vi "Acquire channel.vi"(8 "error in (no error)":errorcluster, 9 "Channel":i32, 10 "Acquisition cluster":T2, 11 "Instrument cluster":T1) -> (0 "error out":errorcluster, 2 "Image Array":u16[][](array[numeric]))   [LabVIEW 2017]
uses:
  C:/Program Files/National Instruments/LabVIEW 2017/instr.lib/IDS/ueye.NET/uEyeDotNet.dll
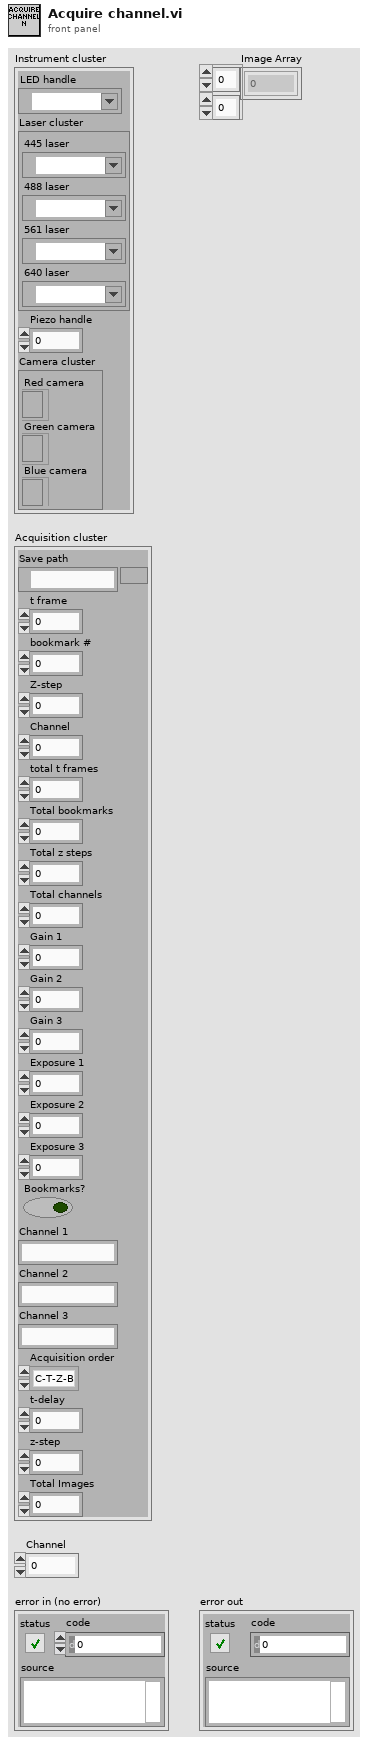
[diagram p1: front panel]
types:
  T1 = cluster{"LED handle":refnum<visa-resource-name>, "Laser cluster":cluster{"445 laser":refnum<visa-resource-name>, "488 laser":refnum<visa-resource-name>, "561 laser":refnum<visa-resource-name>, "640 laser":refnum<visa-resource-name>}, "Piezo handle":i32, "Camera cluster":cluster{"Red camera":refnum<k24>, "Green camera":refnum<k24>, "Blue camera":refnum<k24>}}
  T2 = cluster{"Save path":path, "t frame":i32, "bookmark #":i32, "Z-step":i32, "Channel":i32, "total t frames":i32, "Total bookmarks":i32, "Total z steps":i32, "Total channels":i32, "Gain 1":i32, "Gain 2":i32, "Gain 3":i32, "Exposure 1":dbl, "Exposure 2":dbl, "Exposure 3":dbl, "Bookmarks?":bool, "Channel 1":string, "Channel 2":string, "Channel 3":string, "Acquisition order":enum16{"C-T-Z-B", "C-T-B-Z", "C-Z-T-B", "C-Z-B-T", "C-B-T-Z", "C-B-Z-T", "T-C-Z-B", "T-C-B-Z", "T-Z-C-B", "T-Z-B-C", "T-B-C-Z", "T-B-Z-C", "Z-C-T-B", "Z-C-B-T", "Z-T-C-B", "Z-T-B-C", "Z-B-C-T", "Z-B-T-C", "B-C-T-Z", "B-C-Z-T", "B-Z-C-T", "B-Z-T-C", "B-T-C-Z", "B-T-Z-C"}, "t-delay":dbl, "z-step":dbl, "Total Images":i32}
  T3 = cluster{"445 laser":refnum<visa-resource-name>, "488 laser":refnum<visa-resource-name>, "561 laser":refnum<visa-resource-name>, "640 laser":refnum<visa-resource-name>}
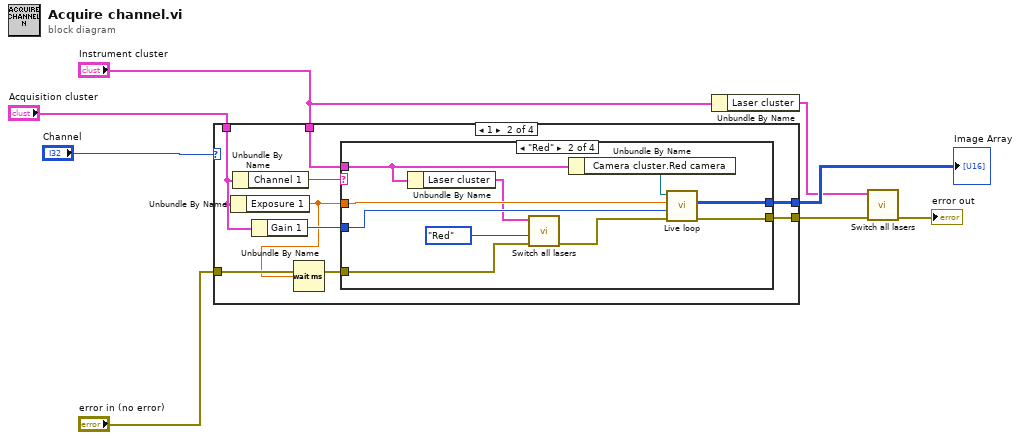
[diagram p0: block diagram]
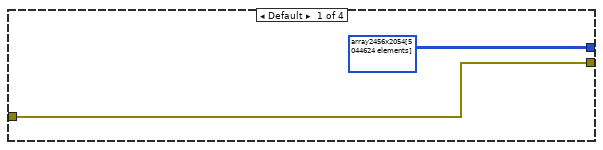
[diagram p2: hidden frame]
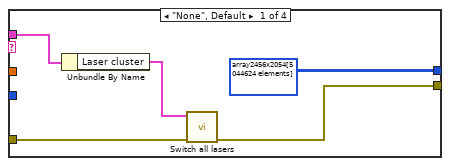
[diagram p3: hidden frame]
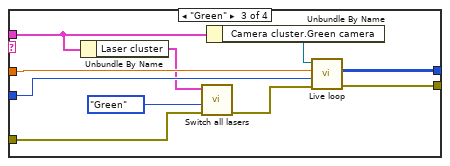
[diagram p4: hidden frame]
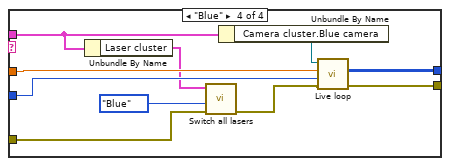
[diagram p5: hidden frame]
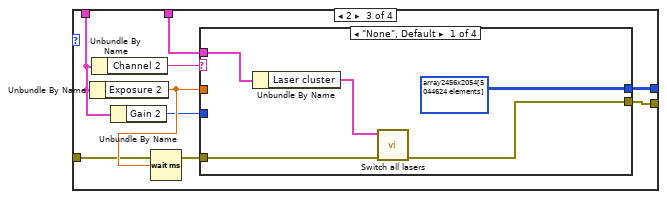
[diagram p6: hidden frame]
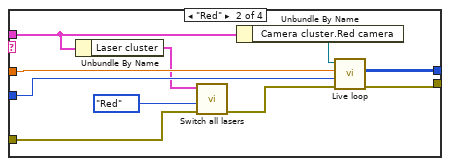
[diagram p7: hidden frame]
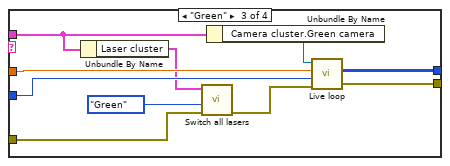
[diagram p8: hidden frame]
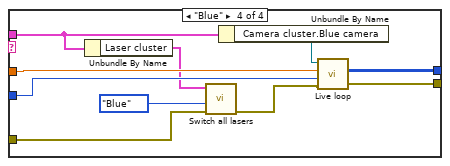
[diagram p9: hidden frame]
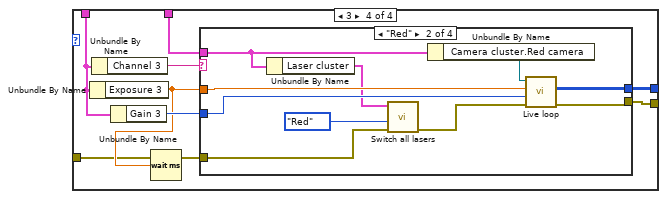
[diagram p10: hidden frame]
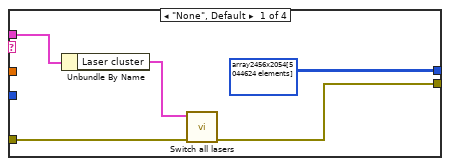
[diagram p11: hidden frame]
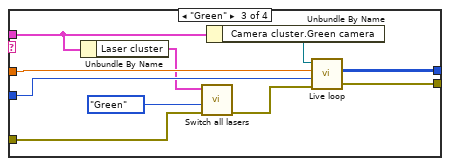
[diagram p12: hidden frame]
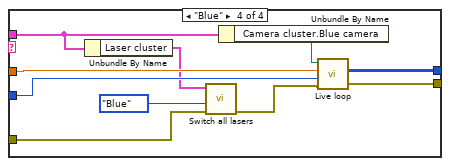
[diagram p13: hidden frame]
diagram:
  n1 = case shown="1" "Channel" {
    tunnel: "Acquisition cluster" -> [_ w17 w61 w104]
    tunnel: "Instrument cluster" -> [_ w16 w59 w101]
    tunnel: "error in (no error)" -> [w10 w14 w55 w97]
    tunnel: [w10 w12 w60 w103] -> w4
    tunnel: [u16[][] array2456x2054[5044624 elements] ("Image Array") w11 w54 w102] -> w6
    frame Default {
    }
    frame 1 {
      n2 = Unbundle By Name(w17) -> ("Exposure 1"=w13:dbl)
      n3 = Unbundle By Name(w17) -> ("Channel 1"=w18:string)
      n4 = Unbundle By Name(w17) -> ("Gain 1"=w15:i32)
      n5 = Wait (ms)(milliseconds to wait=w13) -> ()  [unwired: 1 out]
      n6 = case shown="\"Red\"" w18 {
        tunnel: w16 -> [w19 w25 w36 w45]
        tunnel: w15 -> [_ w33 w43 w53]
        tunnel: w13 -> [_ w32 w42 w52]
        tunnel: w14 -> [w21 w28 w35 w44]
        tunnel: [w20 w29 w39 w49] -> w12
        tunnel: [u16[][] array2456x2054[5044624 elements] ("Image Array") w30 w40 w50] -> w11
        frame "None", Default {
          n7 = Unbundle By Name(w19) -> ("Laser cluster"=w22:T3)
          n8 = call "Switch all lasers.vi"("error in"=w21, "Laser cluster"=w22) -> ("error out"=w20:errorcluster)  [unwired: 9 in]
        }
        frame "Red" {
          n9 = Unbundle By Name(w25) -> ("Laser cluster"=w24:T3)
          n10 = call "Switch all lasers.vi"("error in"=w28, "Live channel"=enum8{"Red", "Green", "Blue", ""}."Red", "Laser cluster"=w24) -> ("error out"=w27:errorcluster)  [unwired: 8 in]
          n11 = Unbundle By Name(w25) -> ("Camera cluster.Red camera"=w31:refnum<k24>)
          n12 = call "Live loop.vi"("Error In"=w27, "Gain"=w33, "Exposure time (ms)"=w32, "Camera reference in"=w31) -> ("Error Out"=w29:errorcluster, "Image Array"=w30:u16[][])  [unwired: 4 in, 1 out]
        }
        frame "Green" {
          n13 = Unbundle By Name(w36) -> ("Laser cluster"=w38:T3)
          n14 = call "Switch all lasers.vi"("error in"=w35, "Live channel"=enum8{"Red", "Green", "Blue", ""}."Green", "Laser cluster"=w38) -> ("error out"=w34:errorcluster)  [unwired: 8 in]
          n15 = Unbundle By Name(w36) -> ("Camera cluster.Green camera"=w41:refnum<k24>)
          n16 = call "Live loop.vi"("Error In"=w34, "Gain"=w43, "Exposure time (ms)"=w42, "Camera reference in"=w41) -> ("Error Out"=w39:errorcluster, "Image Array"=w40:u16[][])  [unwired: 4 in, 1 out]
        }
        frame "Blue" {
          n17 = Unbundle By Name(w45) -> ("Laser cluster"=w48:T3)
          n18 = call "Switch all lasers.vi"("error in"=w44, "Live channel"=enum8{"Red", "Green", "Blue", ""}."Blue", "Laser cluster"=w48) -> ("error out"=w46:errorcluster)  [unwired: 8 in]
          n19 = Unbundle By Name(w45) -> ("Camera cluster.Blue camera"=w51:refnum<k24>)
          n20 = call "Live loop.vi"("Error In"=w46, "Gain"=w53, "Exposure time (ms)"=w52, "Camera reference in"=w51) -> ("Error Out"=w49:errorcluster, "Image Array"=w50:u16[][])  [unwired: 4 in, 1 out]
        }
      }
    }
    frame 2 {
      n21 = Unbundle By Name(w61) -> ("Exposure 2"=w57:dbl)
      n22 = Unbundle By Name(w61) -> ("Channel 2"=w58:string)
      n23 = Unbundle By Name(w61) -> ("Gain 2"=w56:i32)
      n24 = Wait (ms)(milliseconds to wait=w57) -> ()  [unwired: 1 out]
      n25 = case shown="\"None\", Default" w58 {
        tunnel: w59 -> [w62 w68 w79 w88]
        tunnel: w56 -> [_ w76 w86 w96]
        tunnel: w57 -> [_ w75 w85 w95]
        tunnel: w55 -> [w64 w71 w78 w87]
        tunnel: [w63 w72 w82 w92] -> w60
        tunnel: [u16[][] array2456x2054[5044624 elements] ("Image Array") w73 w83 w93] -> w54
        frame "None", Default {
          n26 = Unbundle By Name(w62) -> ("Laser cluster"=w65:T3)
          n27 = call "Switch all lasers.vi"("error in"=w64, "Laser cluster"=w65) -> ("error out"=w63:errorcluster)  [unwired: 9 in]
        }
        frame "Red" {
          n28 = Unbundle By Name(w68) -> ("Laser cluster"=w67:T3)
          n29 = call "Switch all lasers.vi"("error in"=w71, "Live channel"=enum8{"Red", "Green", "Blue", ""}."Red", "Laser cluster"=w67) -> ("error out"=w70:errorcluster)  [unwired: 8 in]
          n30 = Unbundle By Name(w68) -> ("Camera cluster.Red camera"=w74:refnum<k24>)
          n31 = call "Live loop.vi"("Error In"=w70, "Gain"=w76, "Exposure time (ms)"=w75, "Camera reference in"=w74) -> ("Error Out"=w72:errorcluster, "Image Array"=w73:u16[][])  [unwired: 4 in, 1 out]
        }
        frame "Green" {
          n32 = Unbundle By Name(w79) -> ("Laser cluster"=w81:T3)
          n33 = call "Switch all lasers.vi"("error in"=w78, "Live channel"=enum8{"Red", "Green", "Blue", ""}."Green", "Laser cluster"=w81) -> ("error out"=w77:errorcluster)  [unwired: 8 in]
          n34 = Unbundle By Name(w79) -> ("Camera cluster.Green camera"=w84:refnum<k24>)
          n35 = call "Live loop.vi"("Error In"=w77, "Gain"=w86, "Exposure time (ms)"=w85, "Camera reference in"=w84) -> ("Error Out"=w82:errorcluster, "Image Array"=w83:u16[][])  [unwired: 4 in, 1 out]
        }
        frame "Blue" {
          n36 = Unbundle By Name(w88) -> ("Laser cluster"=w91:T3)
          n37 = call "Switch all lasers.vi"("error in"=w87, "Live channel"=enum8{"Red", "Green", "Blue", ""}."Blue", "Laser cluster"=w91) -> ("error out"=w89:errorcluster)  [unwired: 8 in]
          n38 = Unbundle By Name(w88) -> ("Camera cluster.Blue camera"=w94:refnum<k24>)
          n39 = call "Live loop.vi"("Error In"=w89, "Gain"=w96, "Exposure time (ms)"=w95, "Camera reference in"=w94) -> ("Error Out"=w92:errorcluster, "Image Array"=w93:u16[][])  [unwired: 4 in, 1 out]
        }
      }
    }
    frame 3 {
      n40 = Unbundle By Name(w104) -> ("Exposure 3"=w98:dbl)
      n41 = Unbundle By Name(w104) -> ("Channel 3"=w100:string)
      n42 = Unbundle By Name(w104) -> ("Gain 3"=w99:i32)
      n43 = Wait (ms)(milliseconds to wait=w98) -> ()  [unwired: 1 out]
      n44 = case shown="\"Red\"" w100 {
        tunnel: w101 -> [w105 w111 w122 w131]
        tunnel: w99 -> [_ w119 w129 w139]
        tunnel: w98 -> [_ w118 w128 w138]
        tunnel: w97 -> [w107 w114 w121 w130]
        tunnel: [w106 w115 w125 w135] -> w103
        tunnel: [u16[][] array2456x2054[5044624 elements] ("Image Array") w116 w126 w136] -> w102
        frame "None", Default {
          n45 = Unbundle By Name(w105) -> ("Laser cluster"=w108:T3)
          n46 = call "Switch all lasers.vi"("error in"=w107, "Laser cluster"=w108) -> ("error out"=w106:errorcluster)  [unwired: 9 in]
        }
        frame "Red" {
          n47 = Unbundle By Name(w111) -> ("Laser cluster"=w110:T3)
          n48 = call "Switch all lasers.vi"("error in"=w114, "Live channel"=enum8{"Red", "Green", "Blue", ""}."Red", "Laser cluster"=w110) -> ("error out"=w113:errorcluster)  [unwired: 8 in]
          n49 = Unbundle By Name(w111) -> ("Camera cluster.Red camera"=w117:refnum<k24>)
          n50 = call "Live loop.vi"("Error In"=w113, "Gain"=w119, "Exposure time (ms)"=w118, "Camera reference in"=w117) -> ("Error Out"=w115:errorcluster, "Image Array"=w116:u16[][])  [unwired: 4 in, 1 out]
        }
        frame "Green" {
          n51 = Unbundle By Name(w122) -> ("Laser cluster"=w124:T3)
          n52 = call "Switch all lasers.vi"("error in"=w121, "Live channel"=enum8{"Red", "Green", "Blue", ""}."Green", "Laser cluster"=w124) -> ("error out"=w120:errorcluster)  [unwired: 8 in]
          n53 = Unbundle By Name(w122) -> ("Camera cluster.Green camera"=w127:refnum<k24>)
          n54 = call "Live loop.vi"("Error In"=w120, "Gain"=w129, "Exposure time (ms)"=w128, "Camera reference in"=w127) -> ("Error Out"=w125:errorcluster, "Image Array"=w126:u16[][])  [unwired: 4 in, 1 out]
        }
        frame "Blue" {
          n55 = Unbundle By Name(w131) -> ("Laser cluster"=w134:T3)
          n56 = call "Switch all lasers.vi"("error in"=w130, "Live channel"=enum8{"Red", "Green", "Blue", ""}."Blue", "Laser cluster"=w134) -> ("error out"=w132:errorcluster)  [unwired: 8 in]
          n57 = Unbundle By Name(w131) -> ("Camera cluster.Blue camera"=w137:refnum<k24>)
          n58 = call "Live loop.vi"("Error In"=w132, "Gain"=w139, "Exposure time (ms)"=w138, "Camera reference in"=w137) -> ("Error Out"=w135:errorcluster, "Image Array"=w136:u16[][])  [unwired: 4 in, 1 out]
        }
      }
    }
  }
  "Image Array" <- w6
  n59 = Unbundle By Name("Instrument cluster") -> ("Laser cluster"=w1:T3)
  n60 = call "Switch all lasers.vi"("error in"=w4, "Laser cluster"=w1) -> ("error out"=→"error out":errorcluster)  [unwired: 9 in]
